vi "NewPort_PM_USB_OpenDevice(SubVI).vi"(8 "error in":errorcluster) -> (0 "error out":errorcluster, 3 "reference Out":refnum<k24>)   [LabVIEW 2017]
uses:
  C:/Program Files (x86)/Newport/Newport USB Driver/Bin/UsbDllWrap.dll
  Program Files (x86)/Newport/Newport USB Driver/Bin/UsbDllWrap.dll
panel:
  # "Built upon Newport Power Meter USB Driver v4.2.1"
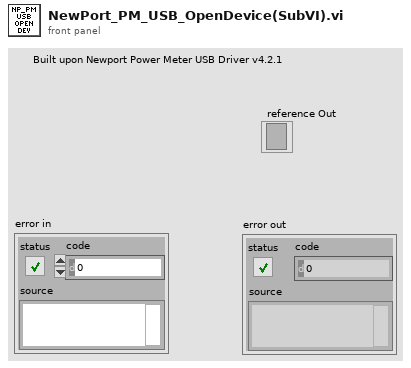
[diagram p1: front panel]
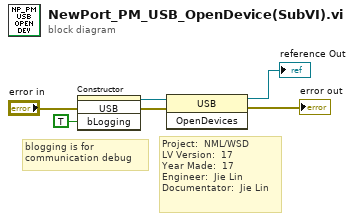
[diagram p0: block diagram]
diagram:
  # "Project:  NML/WSD \nLV Version:  17\nYear Made:  17\nEngineer:  Jie Lin\nDocumentator:  Jie Lin"
  # "blogging is for\ncommunication debug"
  n1 = constructor class="USB"(error in="error in", "bLogging"=TRUE) -> (reference out=w6:refnum<k24>, error out=w5:errorcluster)  [unwired: 2 in, 2 out]
  n2 = invoke class="USB" method="OpenDevices"(reference=w6, error in=w5) -> (reference out=→"reference Out":refnum<k24>, error out=→"error out":errorcluster)  [unwired: 1 in, 1 out]
